vi "GEA3 HEWH Heat Pump.vi"(8 "Error In":errorcluster, 10 "ERD Data In":T3[](array[typedef]) {"ERD Number" format="%.0x"}, 11 "GEA3 ERD Data":T1) -> (0 "Error Out":errorcluster, 3 "GEA3 ERD Data Out":T1, 5 "Mix Valve Data":string[][](array[string]))   [LabVIEW 2020]
uses:
  type defs/ERD Read Data Out.ctl
  Type Definitions/GEA3 HEWH ERD Data.ctl
  Type Definitions/GEA3 HEWH Mixing Valve.ctl
  library/GEA2_Toolkit.lvlib
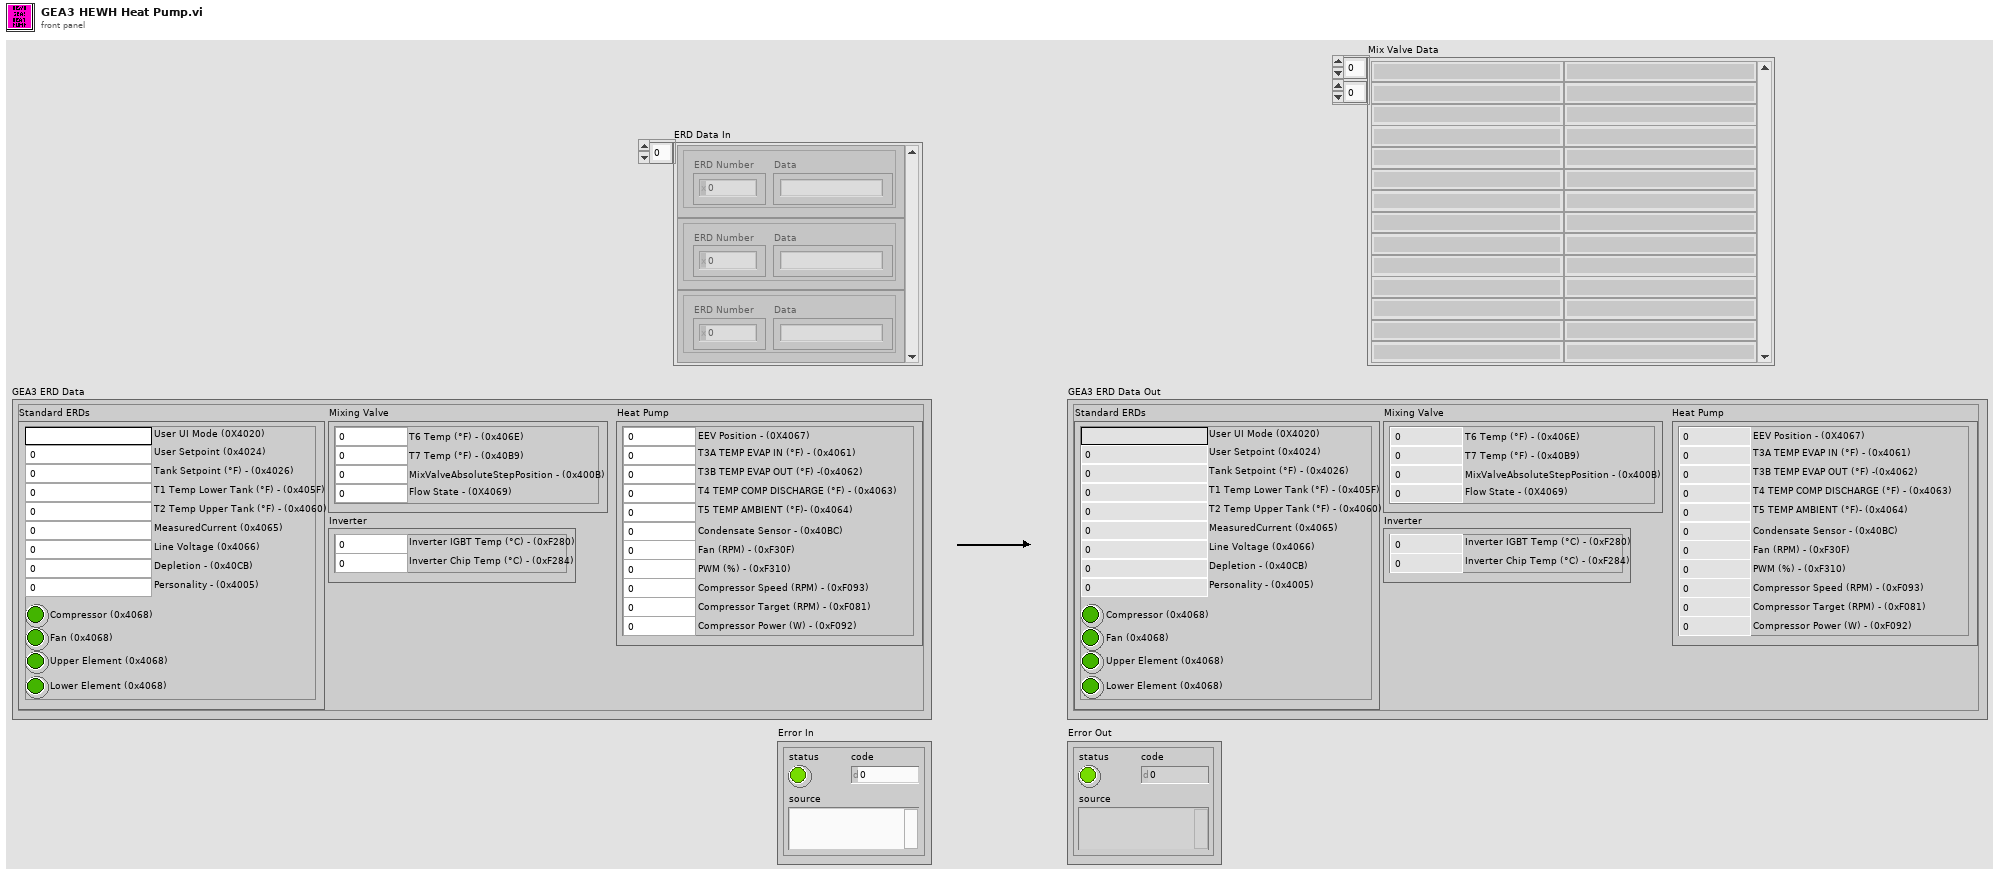
[diagram p1: front panel]
types:
  T1 = typedef "GEA3 HEWH ERD Data.ctl" = cluster{"Mixing Valve":T2, "Standard ERDs":cluster{"User UI Mode (0X4020)":string, "User Setpoint (0x4024)":u16, "Compressor (0x4068)":bool, "Lower Element (0x4068)":bool, "Upper Element (0x4068)":bool, "Fan (0x4068)":bool, "T1 Temp Lower Tank (°F) - (0x405F)":dbl, "T2 Temp Upper Tank (°F) - (0x4060)":dbl, "Line Voltage (0x4066)":u16, "MeasuredCurrent (0x4065)":dbl, "Tank Setpoint (°F) - (0x4026)":u16, "Depletion - (0x40CB)":u16, "Personality - (0x4005)":u16}, "Heat Pump":cluster{"EEV Position - (0X4067)":u16, "T3A TEMP EVAP IN (°F) - (0x4061)":dbl, "T3B TEMP EVAP OUT (°F) -(0x4062)":dbl, "T4 TEMP COMP DISCHARGE (°F) - (0x4063)":dbl, "T5 TEMP AMBIENT (°F)- (0x4064)":dbl, "Condensate Sensor - (0x40BC)":u16, "Fan (RPM) - (0xF30F)":u16, "PWM (%) - (0xF310)":u16, "Compressor Speed (RPM) - (0xF093)":u16, "Compressor Target (RPM) - (0xF081)":u16, "Compressor Power (W) - (0xF092)":u16}, "Inverter":cluster{"Inverter IGBT Temp (°C) - (0xF280)":dbl, "Inverter Chip Temp (°C) - (0xF284)":dbl}}
  T2 = typedef "GEA3 HEWH Mixing Valve.ctl" = cluster{"T7 Temp (°F) - (0x40B9)":dbl, "MixValveAbsoluteStepPosition - (0x400B)":i16, "Flow State - (0X4069)":u8, "T6 Temp (°F) - (0x406E)":dbl}
  T3 = typedef "GEA2_Toolkit.lvlib/ERD Read Data Out.ctl" = cluster{"ERD Number":u16, "Data":string}
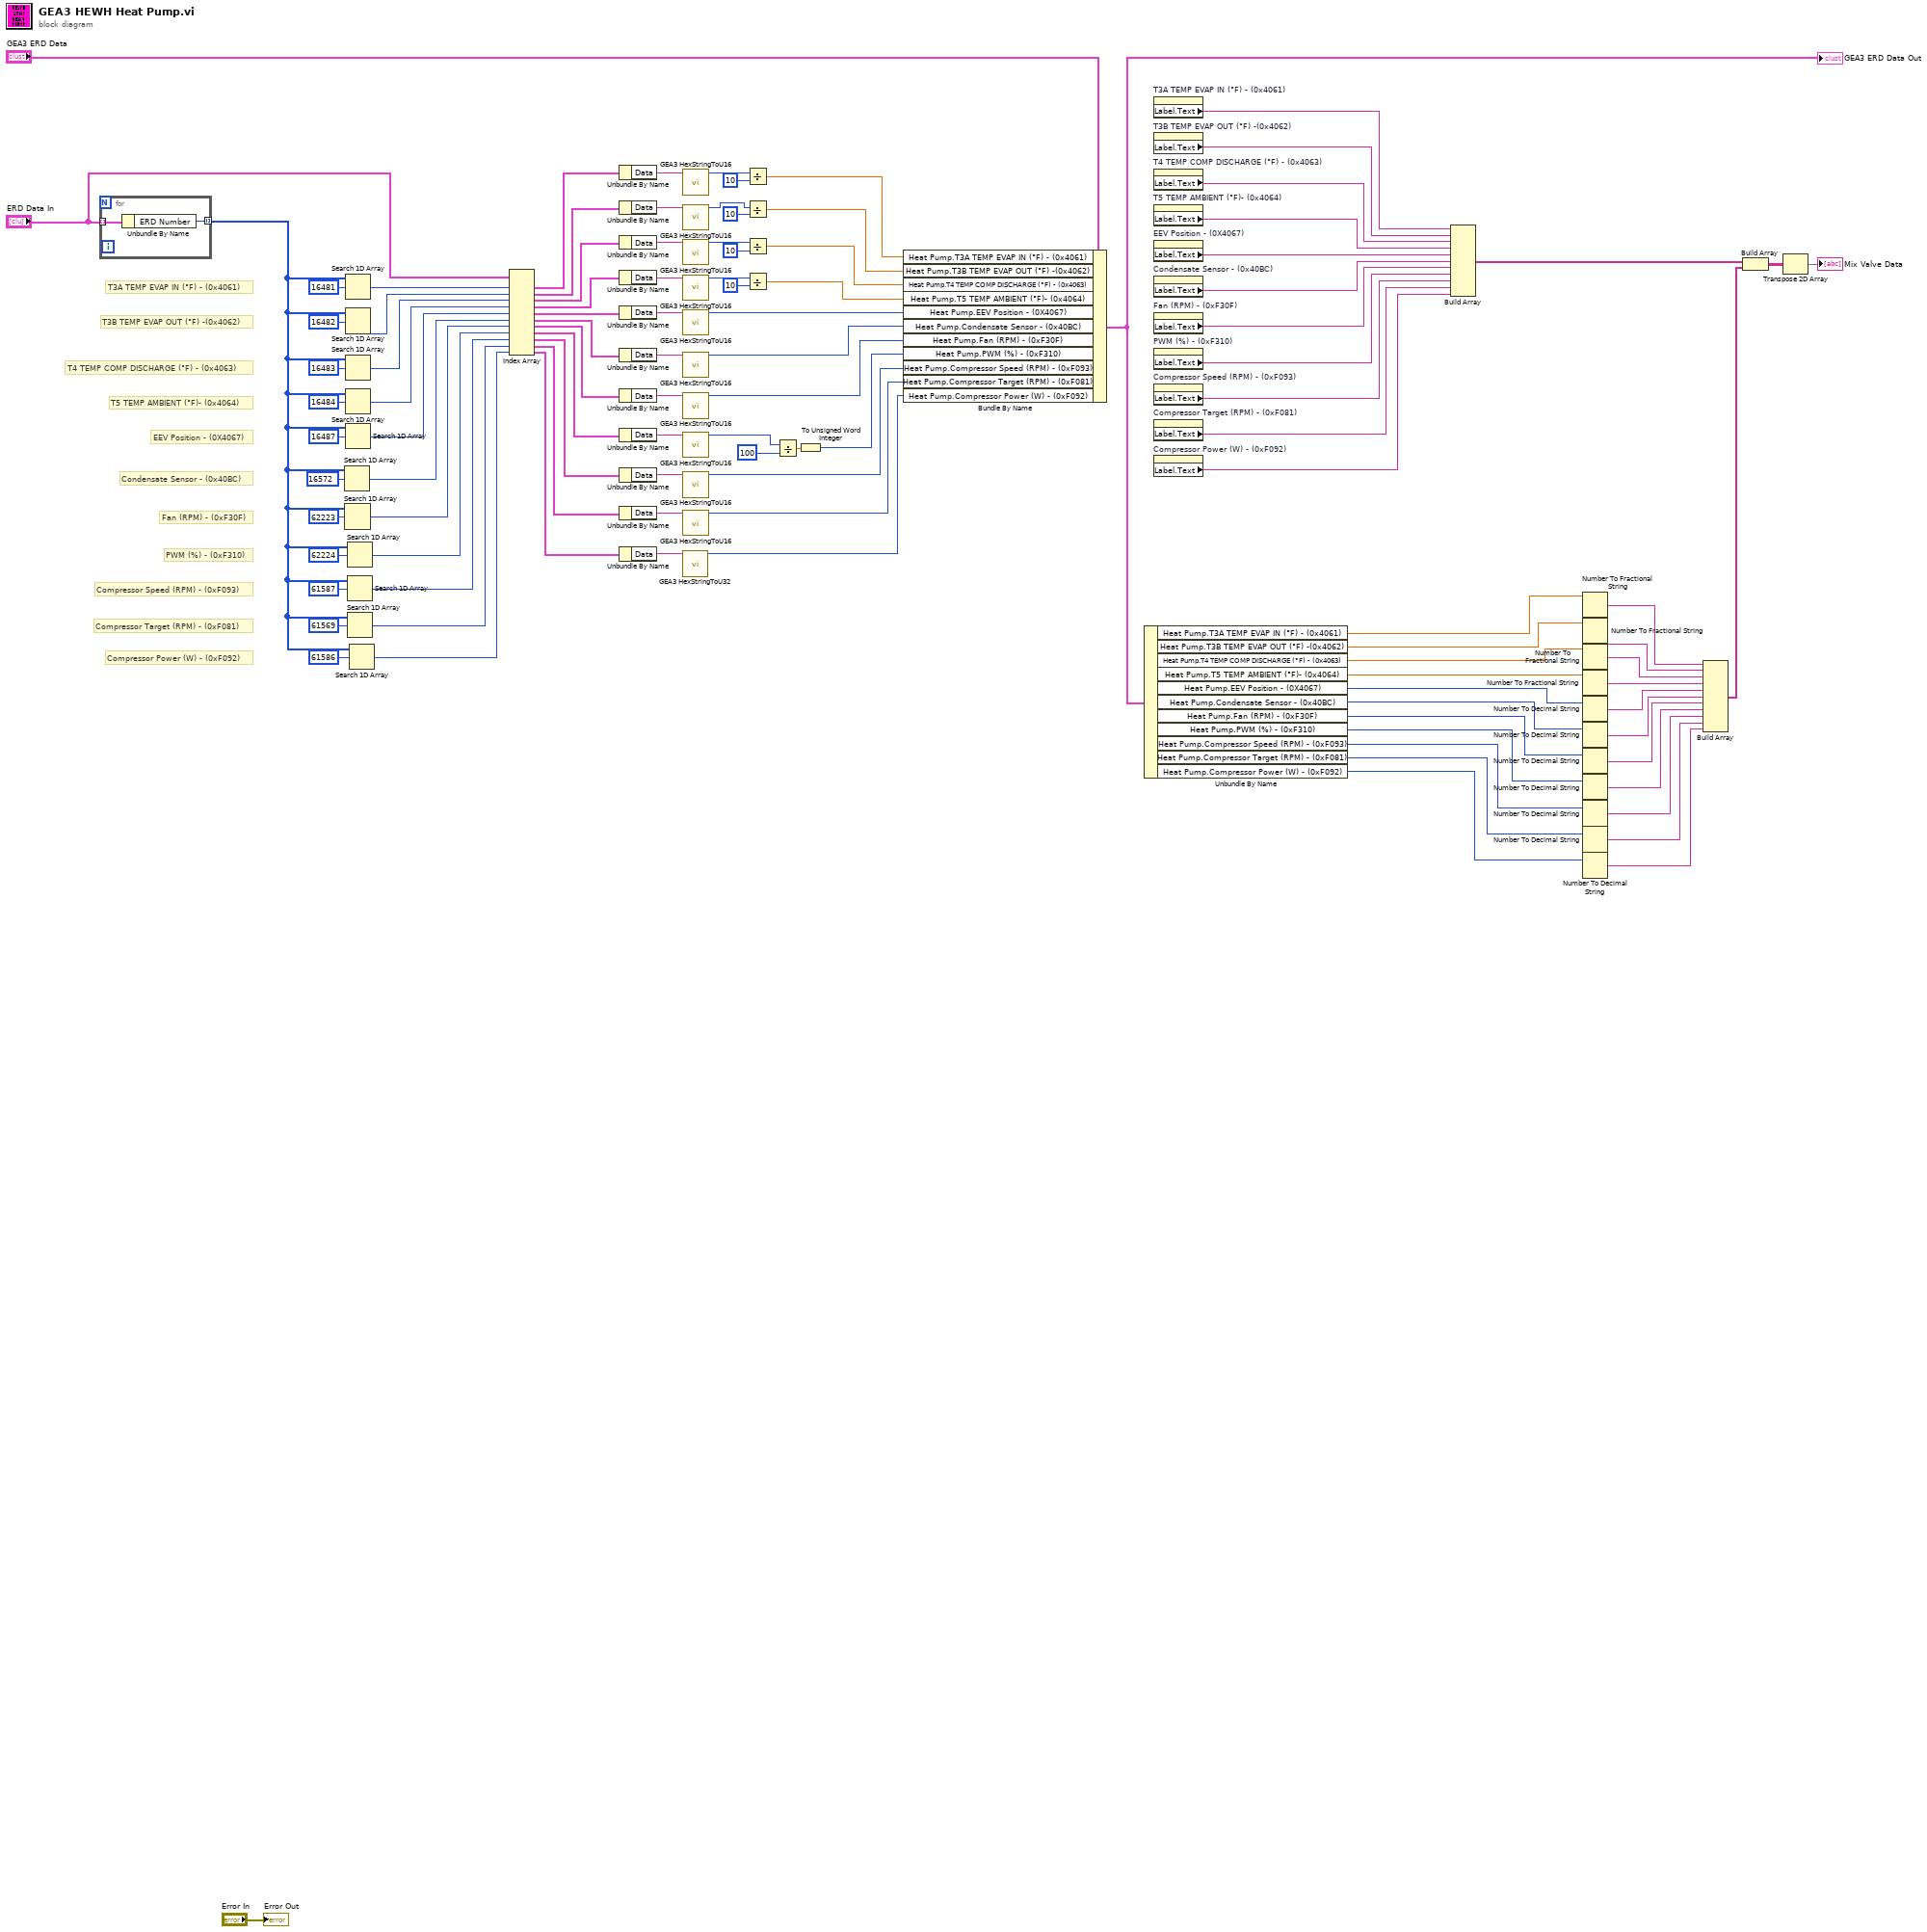
[diagram p0: block diagram]
diagram:
  # "Compressor Power (W) - (0xF092)"
  # "Compressor Target (RPM) - (0xF081)"
  # "Compressor Speed (RPM) - (0xF093)"
  # "PWM (%) - (0xF310)"
  # "Fan (RPM) - (0xF30F)"
  # "Condensate Sensor - (0x40BC)"
  # "T5 TEMP AMBIENT (°F)- (0x4064)"
  # "T4 TEMP COMP DISCHARGE (°F) - (0x4063)"
  # "T3B TEMP EVAP OUT (°F) -(0x4062)"
  # "T3A TEMP EVAP IN (°F) - (0x4061)"
  # "EEV Position - (0X4067)"
  n1 = for {
    tunnel: "ERD Data In" -> [w110] mode=indexing
    tunnel: [w109] -> w46 mode=indexing
    n2 = Unbundle By Name(w110) -> ("ERD Number"=w109:u16)
  }
  n3 = Search 1D Array(1D array=w46, element=u16 16572 ("ERD Number")) -> (index of element=w45:i32)  [unwired: 1 in]
  n4 = Search 1D Array(1D array=w46, element=u16 62223 ("ERD Number")) -> (index of element=w44:i32)  [unwired: 1 in]
  n5 = Search 1D Array(1D array=w46, element=u16 16481 ("ERD Number")) -> (index of element=w89:i32)  [unwired: 1 in]
  n6 = Search 1D Array(1D array=w46, element=u16 16482 ("ERD Number")) -> (index of element=w88:i32)  [unwired: 1 in]
  n7 = Search 1D Array(1D array=w46, element=u16 16483 ("ERD Number")) -> (index of element=w87:i32)  [unwired: 1 in]
  n8 = Search 1D Array(1D array=w46, element=u16 16484 ("ERD Number")) -> (index of element=w86:i32)  [unwired: 1 in]
  n9 = Search 1D Array(1D array=w46, element=u16 16487 ("ERD Number")) -> (index of element=w95:i32)  [unwired: 1 in]
  n10 = Search 1D Array(1D array=w46, element=u16 62224 ("ERD Number")) -> (index of element=w43:i32)  [unwired: 1 in]
  n11 = Search 1D Array(1D array=w46, element=u16 61587 ("ERD Number")) -> (index of element=w42:i32)  [unwired: 1 in]
  n12 = Search 1D Array(1D array=w46, element=u16 61569 ("ERD Number")) -> (index of element=w41:i32)  [unwired: 1 in]
  n13 = Search 1D Array(1D array=w46, element=u16 61586 ("ERD Number")) -> (index of element=w40:i32)  [unwired: 1 in]
  n14 = Index Array(array="ERD Data In", index #1=w89, index #2=w88, index #3=w87, index #4=w86, index #5=w95, index #6=w45, index #7=w44, index #8=w43, index #9=w42, index #10=w41, index #11=w40) -> (element #1=w78:T3, element #2=w79:T3, element #3=w80:T3, element #4=w81:T3, element #5=w94:T3, element #6=w34:T3, element #7=w33:T3, element #8=w32:T3, element #9=w31:T3, element #10=w30:T3, element #11=w29:T3)
  n15 = Unbundle By Name(w78) -> ("Data"=w85:string)
  n16 = Unbundle By Name(w79) -> ("Data"=w84:string)
  n17 = Unbundle By Name(w80) -> ("Data"=w83:string)
  n18 = Unbundle By Name(w81) -> ("Data"=w82:string)
  n19 = Unbundle By Name(w94) -> ("Data"=w106:string)
  n20 = Unbundle By Name(w34) -> ("Data"=w39:string)
  n21 = Unbundle By Name(w33) -> ("Data"=w38:string)
  n22 = Unbundle By Name(w32) -> ("Data"=w37:string)
  n23 = Unbundle By Name(w31) -> ("Data"=w36:string)
  n24 = Unbundle By Name(w30) -> ("Data"=w35:string)
  n25 = Unbundle By Name(w29) -> ("Data"=w6:string)
  n26 = call "GEA3 HexStringToU32.vi"("Input String"=w6) -> ("Number Out"=w5:u32)  [unwired: 14 in]
  n27 = call "GEA3 HexStringToU16.vi"("Input String"=w85) -> ("Number Out"=w76:u16)  [unwired: 14 in]
  n28 = call "GEA3 HexStringToU16.vi"("Input String"=w84) -> ("Number Out"=w72:u16)  [unwired: 14 in]
  n29 = call "GEA3 HexStringToU16.vi"("Input String"=w83) -> ("Number Out"=w71:u16)  [unwired: 14 in]
  n30 = call "GEA3 HexStringToU16.vi"("Input String"=w82) -> ("Number Out"=w70:u16)  [unwired: 14 in]
  n31 = call "GEA3 HexStringToU16.vi"("Input String"=w106) -> ("Number Out"=w105:u16)  [unwired: 14 in]
  n32 = call "GEA3 HexStringToU16.vi"("Input String"=w39) -> ("Number Out"=w28:u16)  [unwired: 14 in]
  n33 = call "GEA3 HexStringToU16.vi"("Input String"=w38) -> ("Number Out"=w27:u16)  [unwired: 14 in]
  n34 = call "GEA3 HexStringToU16.vi"("Input String"=w37) -> ("Number Out"=w3:u16)  [unwired: 14 in]
  n35 = call "GEA3 HexStringToU16.vi"("Input String"=w36) -> ("Number Out"=w26:u16)  [unwired: 14 in]
  n36 = call "GEA3 HexStringToU16.vi"("Input String"=w35) -> ("Number Out"=w25:u16)  [unwired: 14 in]
  n37 = Divide(x=w76, y=u16 10) -> (x/y=w69:dbl)
  n38 = Divide(x=w72, y=u16 10) -> (x/y=w68:dbl)
  n39 = Divide(x=w71, y=u16 10) -> (x/y=w67:dbl)
  n40 = Divide(x=w70, y=u16 10) -> (x/y=w66:dbl)
  n41 = Divide(x=w3, y=u16 100) -> (x/y=w2:dbl)
  n42 = To Unsigned Word Integer(number=w2) -> (unsigned 16bit integer=w1:u16)
  n43 = Bundle By Name(cluster="GEA3 ERD Data", "Heat Pump.T3A TEMP EVAP IN (°F) - (0x4061)"=w69, "Heat Pump.T3B TEMP EVAP OUT (°F) -(0x4062)"=w68, "Heat Pump.T4 TEMP COMP DISCHARGE (°F) - (0x4063)"=w67, "Heat Pump.T5 TEMP AMBIENT (°F)- (0x4064)"=w66, "Heat Pump.EEV Position - (0X4067)"=w105, "Heat Pump.Condensate Sensor - (0x40BC)"=w28, "Heat Pump.Fan (RPM) - (0xF30F)"=w27, "Heat Pump.PWM (%) - (0xF310)"=w1, "Heat Pump.Compressor Speed (RPM) - (0xF093)"=w26, "Heat Pump.Compressor Target (RPM) - (0xF081)"=w25, "Heat Pump.Compressor Power (W) - (0xF092)"=w5) -> (w103:T1)
  "GEA3 ERD Data Out" <- w103
  n44 = Unbundle By Name(w103) -> ("Heat Pump.T3A TEMP EVAP IN (°F) - (0x4061)"=w65:dbl, "Heat Pump.T3B TEMP EVAP OUT (°F) -(0x4062)"=w64:dbl, "Heat Pump.T4 TEMP COMP DISCHARGE (°F) - (0x4063)"=w63:dbl, "Heat Pump.T5 TEMP AMBIENT (°F)- (0x4064)"=w62:dbl, "Heat Pump.EEV Position - (0X4067)"=w102:u16, "Heat Pump.Condensate Sensor - (0x40BC)"=w24:u16, "Heat Pump.Fan (RPM) - (0xF30F)"=w23:u16, "Heat Pump.PWM (%) - (0xF310)"=w22:u16, "Heat Pump.Compressor Speed (RPM) - (0xF093)"=w21:u16, "Heat Pump.Compressor Target (RPM) - (0xF081)"=w20:u16, "Heat Pump.Compressor Power (W) - (0xF092)"=w19:u16)
  n45 = property on="T3A TEMP EVAP IN (°F) - (0x4061)" class="DigNum (strict)"() -> ("Label.Text"=w53:string)  [unwired: 2 in, 2 out]
  n46 = property on="T3B TEMP EVAP OUT (°F) -(0x4062)" class="DigNum (strict)"() -> ("Label.Text"=w54:string)  [unwired: 2 in, 2 out]
  n47 = property on="T4 TEMP COMP DISCHARGE (°F) - (0x4063)" class="DigNum (strict)"() -> ("Label.Text"=w55:string)  [unwired: 2 in, 2 out]
  n48 = property on="T5 TEMP AMBIENT (°F)- (0x4064)" class="DigNum (strict)"() -> ("Label.Text"=w56:string)  [unwired: 2 in, 2 out]
  n49 = property on="EEV Position - (0X4067)" class="DigNum (strict)"() -> ("Label.Text"=w57:string)  [unwired: 2 in, 2 out]
  n50 = property on="Condensate Sensor - (0x40BC)" class="DigNum (strict)"() -> ("Label.Text"=w12:string)  [unwired: 2 in, 2 out]
  n51 = property on="Fan (RPM) - (0xF30F)" class="DigNum (strict)"() -> ("Label.Text"=w11:string)  [unwired: 2 in, 2 out]
  n52 = property on="PWM (%) - (0xF310)" class="DigNum (strict)"() -> ("Label.Text"=w10:string)  [unwired: 2 in, 2 out]
  n53 = property on="Compressor Speed (RPM) - (0xF093)" class="DigNum (strict)"() -> ("Label.Text"=w9:string)  [unwired: 2 in, 2 out]
  n54 = property on="Compressor Target (RPM) - (0xF081)" class="DigNum (strict)"() -> ("Label.Text"=w8:string)  [unwired: 2 in, 2 out]
  n55 = property on="Compressor Power (W) - (0xF092)" class="DigNum (strict)"() -> ("Label.Text"=w7:string)  [unwired: 2 in, 2 out]
  n56 = Build Array(w53, w54, w55, w56, w57, w12, w11, w10, w9, w8, w7) -> (w97:string[])
  n57 = Number To Fractional String(number=w65) -> (F-format string=w61:string)  [unwired: 3 in]
  n58 = Number To Fractional String(number=w64) -> (F-format string=w60:string)  [unwired: 3 in]
  n59 = Number To Fractional String(number=w63) -> (F-format string=w59:string)  [unwired: 3 in]
  n60 = Number To Fractional String(number=w62) -> (F-format string=w58:string)  [unwired: 3 in]
  n61 = Number To Decimal String(number=w102) -> (decimal integer string=w101:string)  [unwired: 1 in]
  n62 = Number To Decimal String(number=w24) -> (decimal integer string=w18:string)  [unwired: 1 in]
  n63 = Number To Decimal String(number=w23) -> (decimal integer string=w17:string)  [unwired: 1 in]
  n64 = Number To Decimal String(number=w22) -> (decimal integer string=w16:string)  [unwired: 1 in]
  n65 = Number To Decimal String(number=w21) -> (decimal integer string=w15:string)  [unwired: 1 in]
  n66 = Number To Decimal String(number=w20) -> (decimal integer string=w14:string)  [unwired: 1 in]
  n67 = Number To Decimal String(number=w19) -> (decimal integer string=w13:string)  [unwired: 1 in]
  n68 = Build Array(w61, w60, w59, w58, w101, w18, w17, w16, w15, w14, w13) -> (w98:string[])
  n69 = Build Array(w97, w98) -> (w100:string[][])
  n70 = Transpose 2D Array(2D array=w100) -> (transposed array=→"Mix Valve Data":string[][])
  "Error Out" <- "Error In"
